vi "RangeFinderCal.vi"() -> ()   [LabVIEW 2014]
uses:
  controls/RangeFind_process.ctl
  controls/ConfigData.ctl
  <vilib>/Instr/_visa.llb/VISA Flush IO Buffer Mask.ctl
  <vilib>/Instr/_visa.llb/VISA Configure Serial Port (Instr).vi
  <vilib>/Utility/file.llb/Write To Spreadsheet File (string).vi
  <vilib>/Analysis/NI_AALBase.lvlib
panel:
  out "Connected":bool
  in  "stop":bool
  in  "Tab Control":T1(tab)
  out "setupEnDisab":bool
  in  "file path (dialog if empty)":path
  in  "Max Range 4":dbl caption="Max Range" format="%.2g"
  in  "Max Range 3":dbl caption="Max Range" format="%.2g"
  in  "Max Range 2":dbl caption="Max Range" format="%.2g"
  in  "Max Range 1":dbl caption="Max Range" format="%.2g"
  in  "Sensor 4 Label":string
  in  "Sensor 3 Label":string
  in  "Sensor 2 Label":string
  in  "Sensor 1 Label":string
  in  "Sample Rate (ms)":dbl=100.0
  in  "Test Name":string
  in  "Connect":bool
  in  "Data System Interface Port":refnum<visa-resource-name>
  out "Range Finder sensor RAW OUTPUT":string
  out "Range Finder sensor parsed output":string[](array[string])
  out "Sensor 4":dbl(slide) caption="Garmin" scale=0.0..200.0
  out "Sensor 3":dbl(slide) caption="HC-SR04" scale=0.0..200.0
  out "Sensor 2":dbl(slide) caption="LidarLite" scale=0.0..200.0
  out "Sensor 1":dbl(slide) caption="SF11-C" scale=0.0..201.0
  in  "Collect":bool
  in  "Comment":string
  out "lblSensor4":string
  out "lblSensor3":string
  out "lblSensor2":string
  out "lblSensor1":string
  in  "Distance":dbl
  out "Mean Sens 4":dbl
  out "S.D. Sensor 4":dbl
  out "Samples":string[][](array[string])
  out "S.D. Sensor 2":dbl
  out "S.D. Sensor 3":dbl
  out "Mean Sens 1":dbl
  out "Mean Sens 2":dbl
  out "Mean Sens 3":dbl
  out "S.D.  Sensor 1":dbl
  in  "writeFile":bool
  out "Activity Log":string
  # ".CSV"
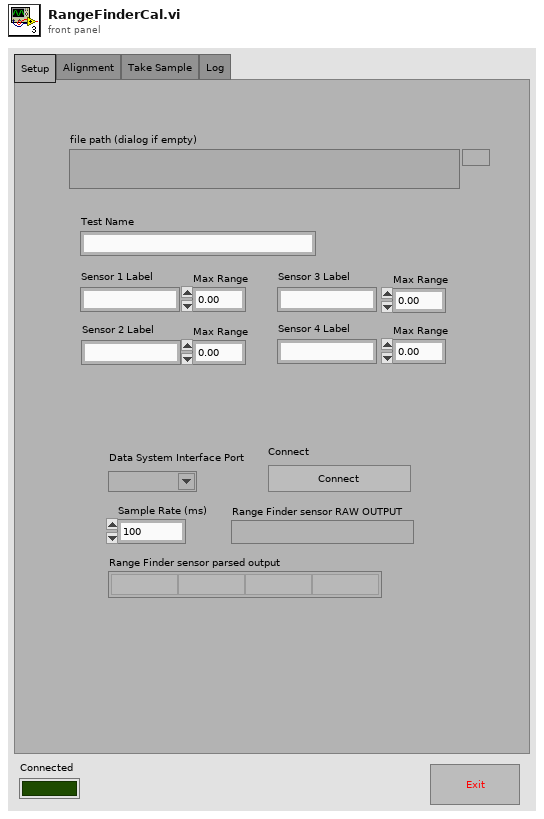
[diagram p1: front panel]
types:
  T1 = enum32{"Setup", "Alignment", "Take Sample", "Log"}
  T2 = typedef "ConfigData.ctl" = cluster{"file path (dialog if empty)":path, "Test Name":string, "Sensor 1 Label":string, "Sensor 2 Label ":string, "Sensor 3 Label":string, "Sensor 4 Label":string, "Max Range":dbl, "Max Range 2":dbl, "Max Range 3":dbl, "Max Range 4":dbl, "Comment":string, "Data System Interface Port":refnum<visa-resource-name>, "Sample Rate":dbl, "error":errorcluster}
  T3 = typedef "RangeFind_process.ctl" = enum16{"Error", "Setup", "Initialize", "Collect", "Store", "Done"}
  T4 = enum8{"Enabled", "Disabled", "Disabled and Grayed Out"}
  T5 = typedef "VISA Flush IO Buffer Mask.ctl" = u16
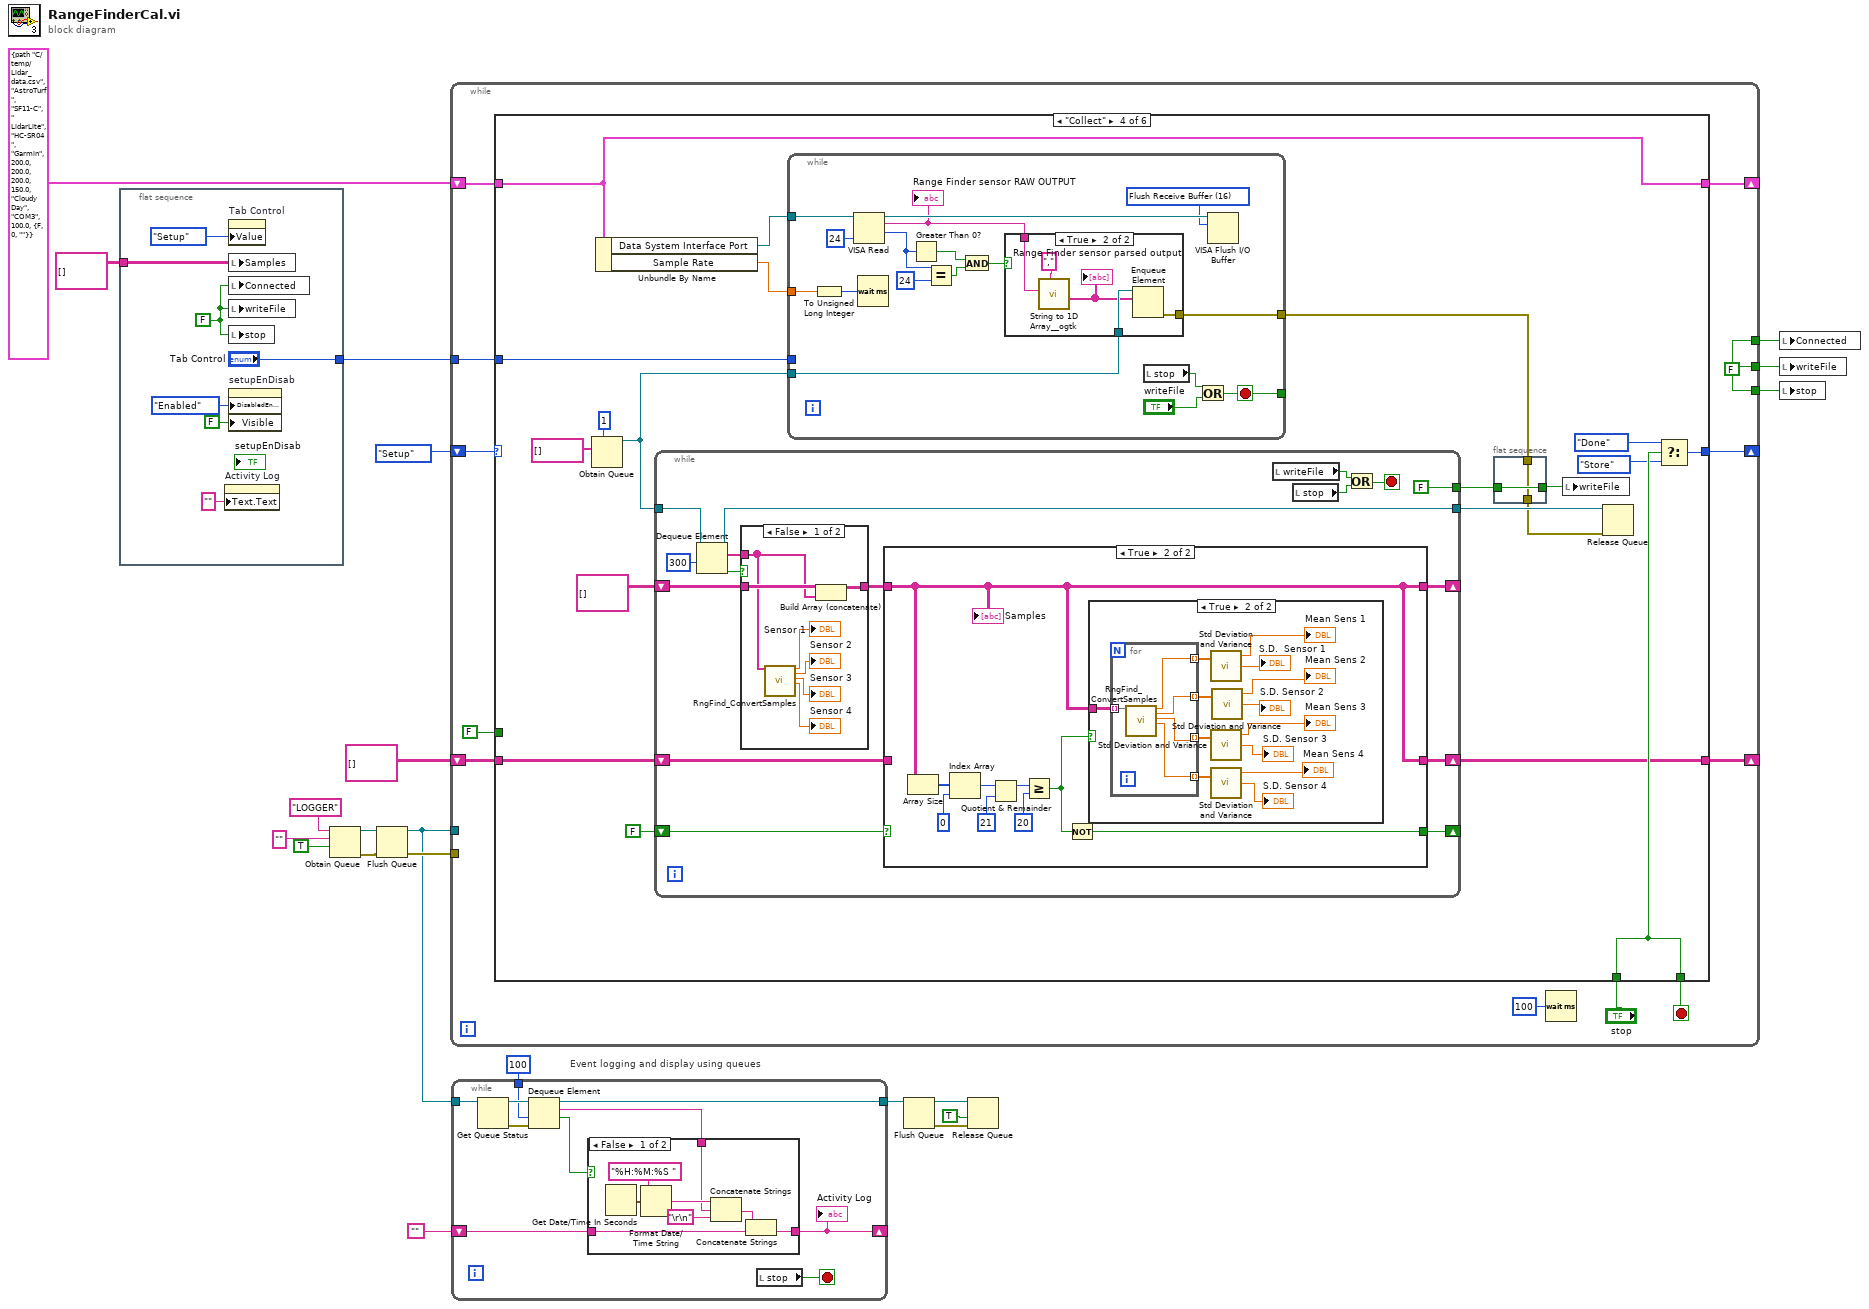
[diagram p0: block diagram]
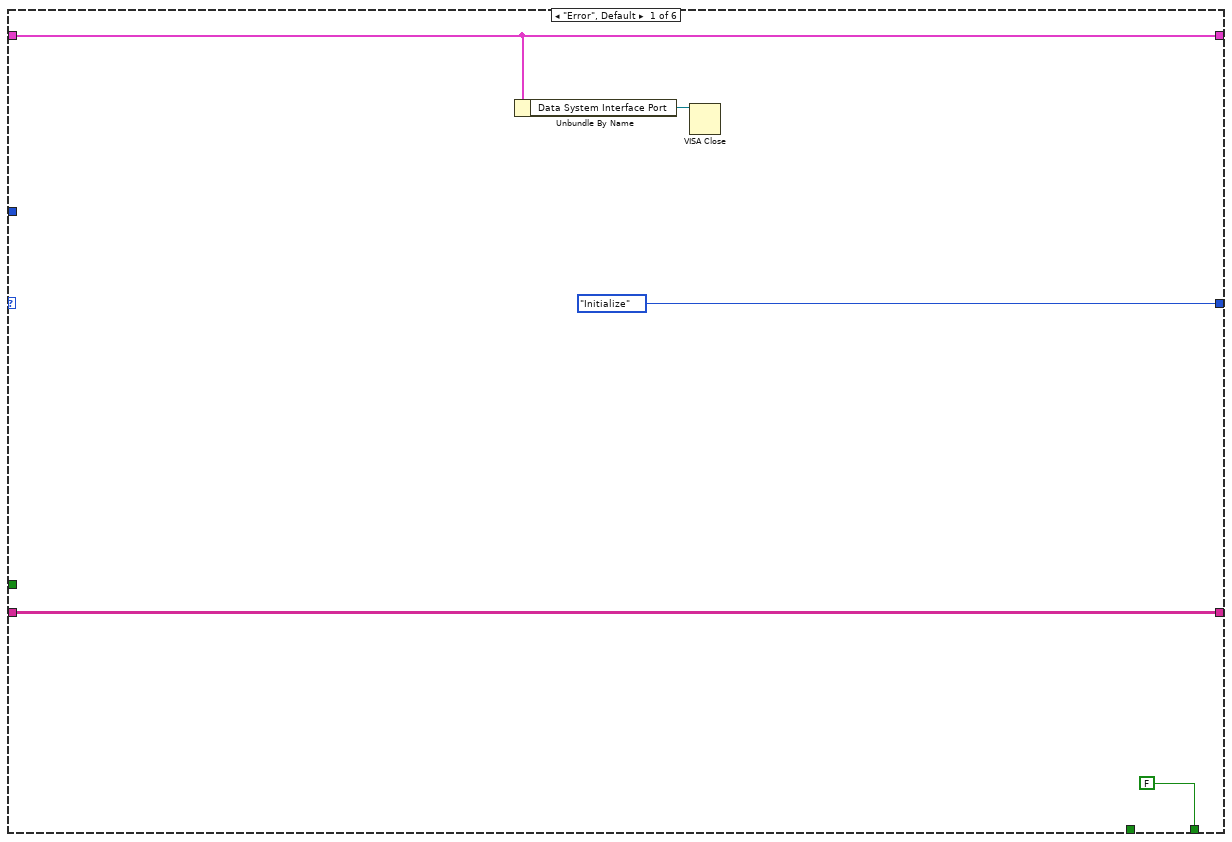
[diagram p3: hidden frame]
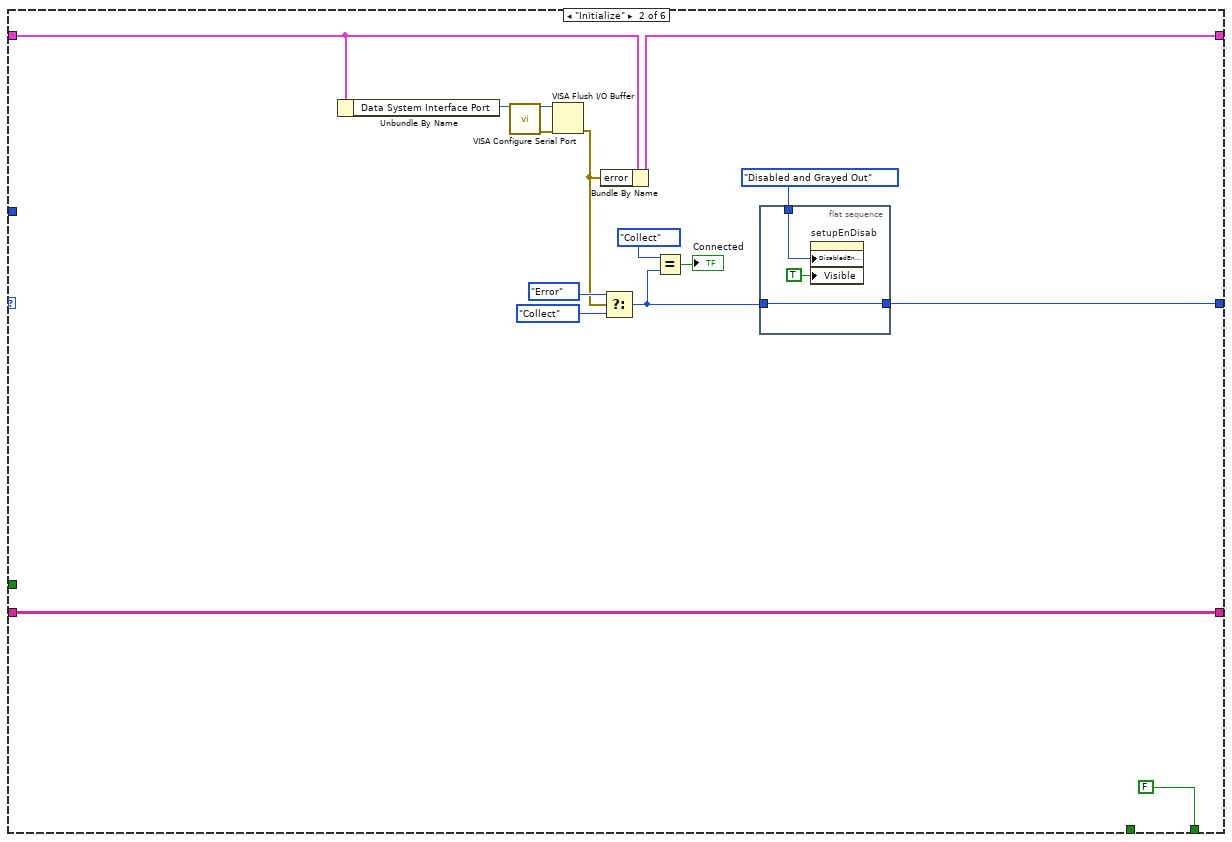
[diagram p4: hidden frame]
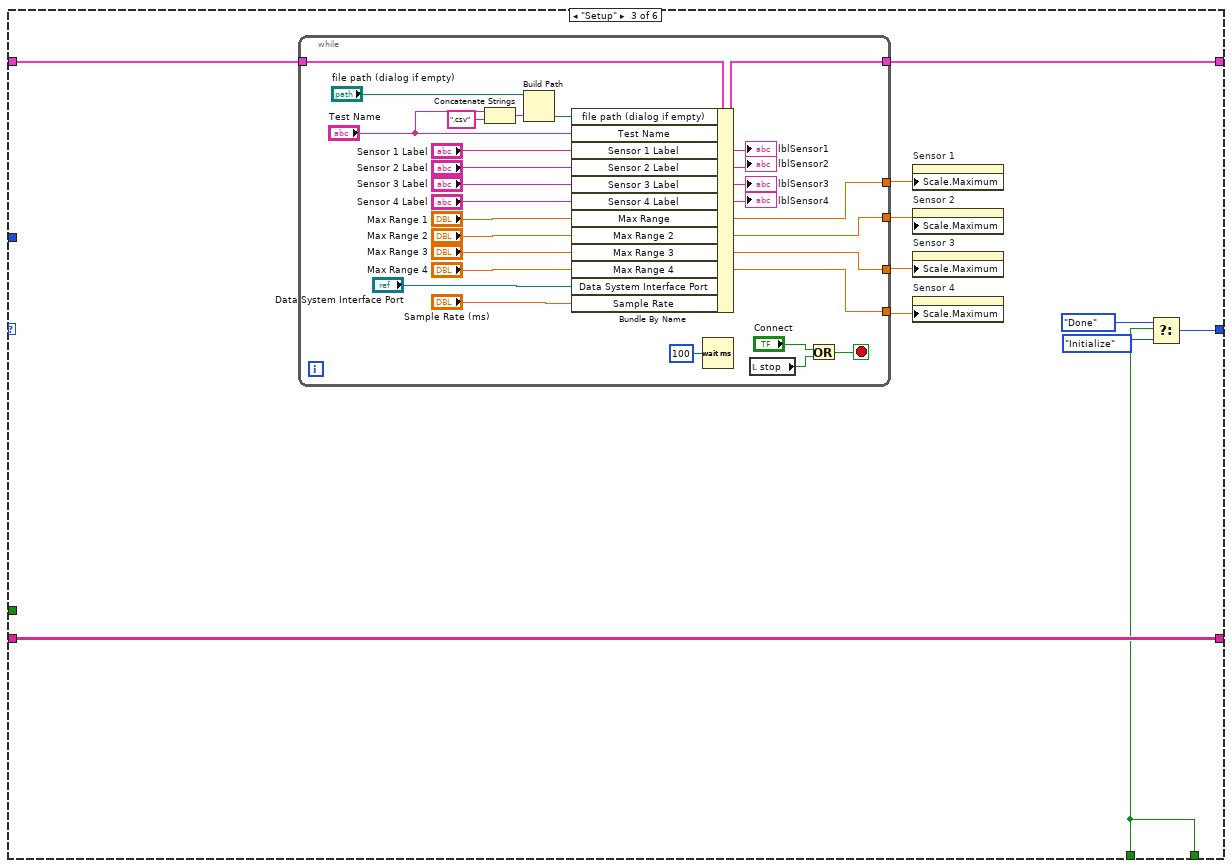
[diagram p5: hidden frame]
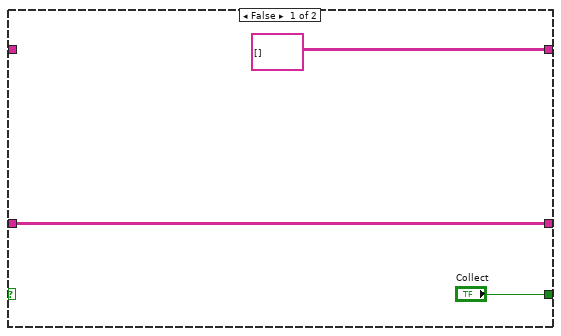
[diagram p6: hidden frame]
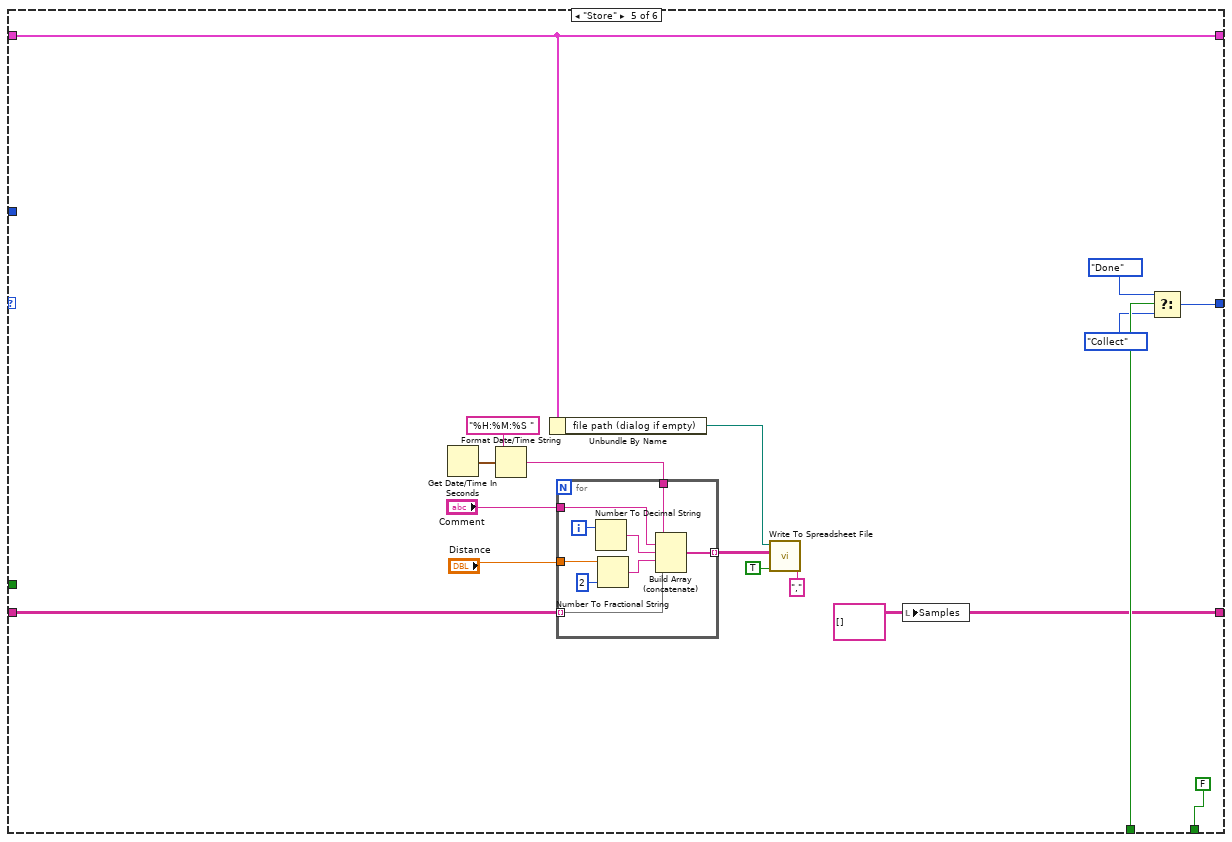
[diagram p10: hidden frame]
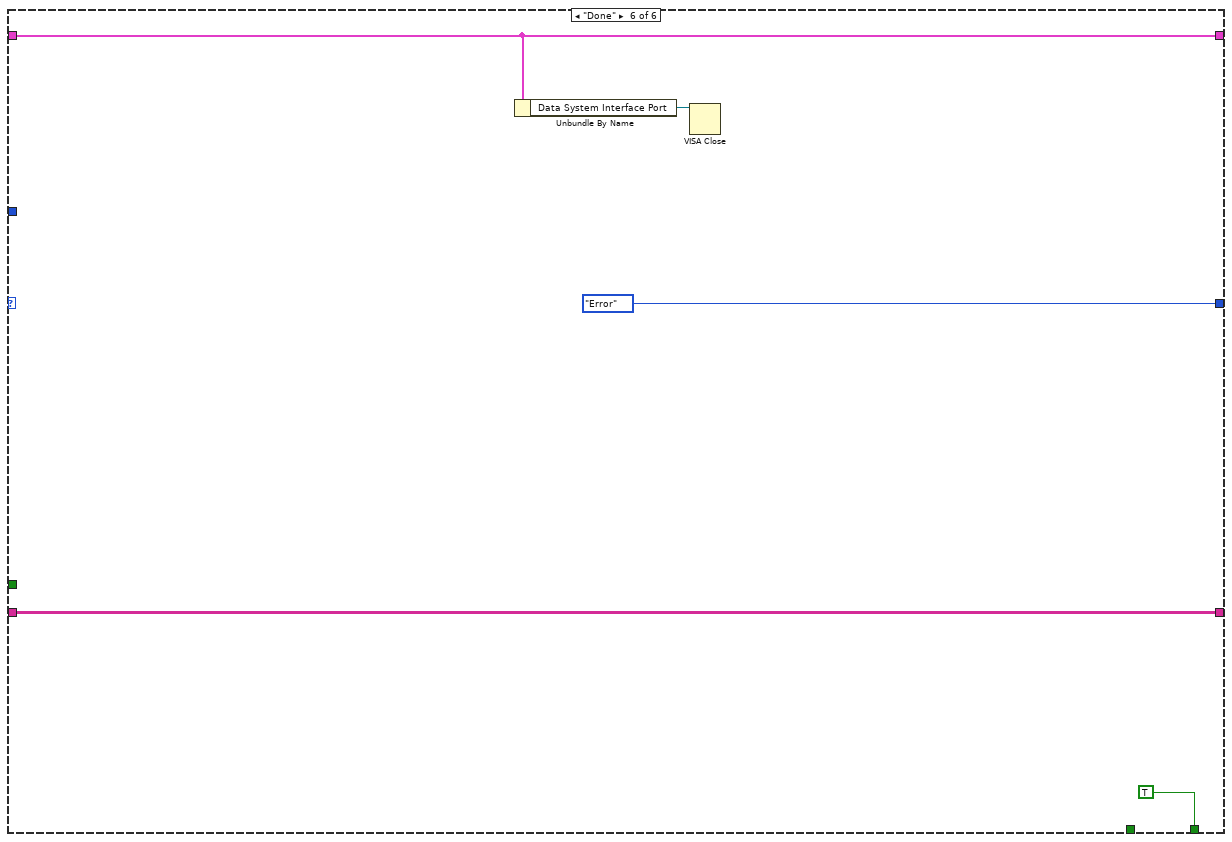
[diagram p11: hidden frame]
diagram:
  # "Event logging and display using queues"
  n1 = flat-sequence {
    tunnel: ["Tab Control"] -> w20
    tunnel: string[][] [] -> [w26]
    frame #0 {
      w25 = FALSE ("stop")
      n2 = property on="Activity Log" class="Str"("Text.Text"="") -> ()  [unwired: 2 in, 2 out]
      n3 = property on="Tab Control" class="TabCtl (strict)"("Value"=T1."Setup" ("Tab Control")) -> ()  [unwired: 2 in, 2 out]
      n4 = local write "Samples"(w26) -> ()
      n5 = local write "Connected"(w25) -> ()
      n6 = local write "writeFile"(w25) -> ()
      n7 = local write "stop"(w25) -> ()
      n8 = property on="setupEnDisab" class="Bool (strict)"("DisabledEnum"=T4."Enabled" ("Disabled"), "Visible"=FALSE) -> ()  [unwired: 2 in, 2 out]
    }
  }
  n9 = Obtain Queue(name (unnamed)="LOGGER", element data type="", create if not found? (T)=TRUE) -> (queue out=w9:refnum<queue>, error out=w13:errorcluster)  [unwired: 2 in, 1 out]
  n10 = Flush Queue(queue=w9) -> (queue out=w3:refnum<queue>)  [unwired: 1 in, 2 out]
  n11 = while {
    tunnel: w20 -> [w39]
    shift-right: [w37] -> _
    shift-left: RangeFind_process."Setup" -> [w38]
    shift-right: [w33] -> _
    shift-left: T2 {"file path (dialog if empty)"=path "C:/temp/Lidar_data.csv", "Test Name"="AstroTurf", "Sensor 1 Label"="SF11-C", "Sensor 2 Label "=" LidarLite", "Sensor 3 Label"="HC-SR04", "Sensor 4 Label"="Garmin", "Max Range"=200.0, "Max Range 2"=200.0, "Max Range 3"=200.0, "Max Range 4"=150.0, "Comment"="Cloudy Day", "Data System Interface Port"="COM3", "Sample Rate"=100.0, "error"={"status"=FALSE, "code"=0, "source"=""}} ("ConfigData") -> [w34]
    shift-right: [w31] -> _
    shift-left: string[][] [] -> [w32]
    tunnel: [w29] -> w16
    tunnel: [w29] -> w15
    tunnel: [w29] -> w14
    tunnel: w13 -> [_]
    tunnel: w3 -> [_]
    stop <- w35 stop-if-true
    w29 = FALSE ("stop")
    n12 = case shown="\"Collect\"" w38 {
      tunnel: w39 -> [_ _ _ w110 _ _]
      tunnel: [RangeFind_process."Initialize" w46 w67 w104 w202 RangeFind_process."Error"] -> w37
      tunnel: [FALSE FALSE w70 w107 FALSE TRUE] -> w35
      tunnel: w34 -> [w40 w52 w73 w108 w207 w219]
      tunnel: [w40 w57 w72 w108 w207 w219] -> w33
      tunnel: w32 -> [w42 w50 w71 w101 w199 w220]
      tunnel: [w42 w50 w71 w103 w200 w220] -> w31
      tunnel: "stop" -> [_ _ w70 w107 w205 _]
      tunnel: FALSE ("stop") -> [_ _ _ _ _ _]
      frame "Error", Default {
        n13 = Unbundle By Name(w40) -> ("Data System Interface Port"=w41:refnum<visa-resource-name>)
        n14 = VISA Close(VISA resource name=w41) -> ()  [unwired: 1 in, 1 out]
      }
      frame "Initialize" {
        n15 = Unbundle By Name(w52) -> ("Data System Interface Port"=w51:refnum<visa-resource-name>)
        n16 = call-poly "VISA Configure Serial Port"("VISA resource name"=w51) -> ("VISA resource name out"=w59:refnum<visa-resource-name>, "error out"=w56:errorcluster)  [unwired: 13 in]
        n17 = VISA Flush I/O Buffer(VISA resource name=w59, error in (no error)=w56) -> (error out=w54:errorcluster)  [unwired: 1 in, 1 out]
        n18 = Bundle By Name(cluster=w52, "error"=w54) -> (w57:T2)
        n19 = Select(t=RangeFind_process."Error", s=w54, f=RangeFind_process."Collect") -> (s? t:f=w47:T3)
        n20 = Equal?(x=RangeFind_process."Collect", y=w47) -> (x = y?=→"Connected":bool)
        n21 = flat-sequence {
          tunnel: w47 -> [w62]
          tunnel: [w62] -> w46
          tunnel: T4."Disabled and Grayed Out" ("Disabled") -> [w60]
          frame #0 {
            n22 = property on="setupEnDisab" class="Bool (strict)"("DisabledEnum"=w60, "Visible"=TRUE) -> ()  [unwired: 2 in, 2 out]
          }
        }
      }
      frame "Setup" {
        n23 = while {
          tunnel: w73 -> [w93]
          tunnel: [w92] -> w72
          tunnel: ["Max Range 1"] -> w66
          tunnel: ["Max Range 2"] -> w65
          tunnel: ["Max Range 3"] -> w64
          tunnel: ["Max Range 4"] -> w63
          stop <- w83 stop-if-true
          n24 = Concatenate Strings("Test Name", ".csv" ("string")) -> (w77:string)
          n25 = Build Path(base path="file path (dialog if empty)", name or relative path=w77) -> (appended path=w76:path)
          n26 = Bundle By Name(cluster=w93, "file path (dialog if empty)"=w76, "Test Name"="Test Name", "Sensor 1 Label"="Sensor 1 Label", "Sensor 2 Label"="Sensor 2 Label", "Sensor 3 Label"="Sensor 3 Label", "Sensor 4 Label"="Sensor 4 Label", "Max Range"="Max Range 1", "Max Range 2"="Max Range 2", "Max Range 3"="Max Range 3", "Max Range 4"="Max Range 4", "Data System Interface Port"="Data System Interface Port", "Sample Rate"="Sample Rate (ms)") -> (w92:T2)
          n27 = Wait (ms)(milliseconds to wait=u32 100) -> ()  [unwired: 1 out]
          n28 = local read "stop"() -> (w84:bool)
          n29 = Or(x="Connect", y=w84) -> (x .or. y?=w83:bool)
          "lblSensor1" <- "Sensor 1 Label"
          "lblSensor2" <- "Sensor 2 Label"
          "lblSensor3" <- "Sensor 3 Label"
          "lblSensor4" <- "Sensor 4 Label"
        }
        n30 = property on="Sensor 1" class="Slide (strict)"("Scale.Maximum"=w66) -> ()  [unwired: 2 in, 2 out]
        n31 = property on="Sensor 2" class="Slide (strict)"("Scale.Maximum"=w65) -> ()  [unwired: 2 in, 2 out]
        n32 = property on="Sensor 3" class="Slide (strict)"("Scale.Maximum"=w64) -> ()  [unwired: 2 in, 2 out]
        n33 = property on="Sensor 4" class="Slide (strict)"("Scale.Maximum"=w63) -> ()  [unwired: 2 in, 2 out]
        n34 = Select(t=RangeFind_process."Done", s=w70, f=RangeFind_process."Initialize") -> (s? t:f=w67:T3)
      }
      frame "Collect" {
        n35 = Obtain Queue(max queue size (-1, unlimited)=1, element data type=string[] []) -> (queue out=w114:refnum<queue>)  [unwired: 3 in, 2 out]
        n36 = Unbundle By Name(w108) -> ("Data System Interface Port"=w109:refnum<visa-resource-name>, "Sample Rate"=w100:dbl)
        n37 = while {
          tunnel: w114 -> [w132]
          tunnel: [w129] -> w112
          shift-right: [w126] -> _
          shift-left: string[][] [] -> [w127]
          tunnel: [FALSE] -> w97
          shift-right: [w119] -> w103
          shift-left: w101 -> [w120]
          shift-right: [w117] -> _
          shift-left: FALSE -> [w118]
          stop <- w121 stop-if-true
          n38 = Dequeue Element(queue=w132, timeout in ms (-1)=300) -> (queue out=w129:refnum<queue>, element=w128:string[], timed out?=w130:bool)  [unwired: 1 in, 1 out]
          n39 = case shown="False" w130 {
            tunnel: w128 -> [w167 _]
            tunnel: w127 -> [w169 w170]
            tunnel: [w168 w170] -> w124
            frame False {
              n40 = call "RngFind_ConvertSamples.vi"("Input Samples"=w167) -> ("sensor 1"=→"Sensor 1":dbl, "sensor 2"=→"Sensor 2":dbl, "sensor 3"=→"Sensor 3":dbl, "sensor 4"=→"Sensor 4":dbl)  [unwired: 15 in]
              n41 = Build Array (concatenate)(w169, w167) -> (w168:string[][])
            }
            frame True {
            }
          }
          n42 = case shown="True" w118 {
            tunnel: [string[][] [] w137] -> w126
            tunnel: w124 -> [_ w137]
            tunnel: w120 -> [w134 _]
            tunnel: [w134 w137] -> w119
            tunnel: ["Collect" w136] -> w117
            frame False {
            }
            frame True {
              n43 = Array Size(array=w137) -> (size(s)=w144:i32[])
              n44 = Index Array(array=w144, index=0) -> (element=w142:i32)
              n45 = Quotient & Remainder(x=w142, y=21) -> (x-y*floor(x/y)=w140:i32)  [unwired: 1 out]
              n46 = Greater Or Equal?(x=w140, y=20) -> (x >= y?=w138:bool)
              n47 = Not(x=w138) -> (.not. x?=w136:bool)
              n48 = case shown="True" w138 {
                tunnel: w137 -> [_ w148]
                frame False {
                }
                frame True {
                  n49 = for {
                    tunnel: w148 -> [w162] mode=indexing
                    tunnel: [w161] -> w157 mode=indexing
                    tunnel: [w158] -> w156 mode=indexing
                    tunnel: [w159] -> w155 mode=indexing
                    tunnel: [w160] -> w147 mode=indexing
                    n50 = call "RngFind_ConvertSamples.vi"("Input Samples"=w162) -> ("sensor 1"=w161:dbl, "sensor 2"=w158:dbl, "sensor 3"=w159:dbl, "sensor 4"=w160:dbl)  [unwired: 15 in]
                  }
                  n51 = call <vilib>:"Std Deviation and Variance.vi"("X"=w157) -> ("mean"=→"Mean Sens 1":dbl, "standard deviation"=→"S.D.  Sensor 1":dbl)  [unwired: 1 in, 1 out]
                  n52 = call <vilib>:"Std Deviation and Variance.vi"("X"=w155) -> ("mean"=→"Mean Sens 3":dbl, "standard deviation"=→"S.D. Sensor 3":dbl)  [unwired: 1 in, 1 out]
                  n53 = call <vilib>:"Std Deviation and Variance.vi"("X"=w147) -> ("mean"=→"Mean Sens 4":dbl, "standard deviation"=→"S.D. Sensor 4":dbl)  [unwired: 1 in, 1 out]
                  n54 = call <vilib>:"Std Deviation and Variance.vi"("X"=w156) -> ("mean"=→"Mean Sens 2":dbl, "standard deviation"=→"S.D. Sensor 2":dbl)  [unwired: 1 in, 1 out]
                }
              }
              "Samples" <- w137
            }
          }
          n55 = local read "writeFile"() -> (w123:bool)
          n56 = local read "stop"() -> (w122:bool)
          n57 = Or(x=w123, y=w122) -> (x .or. y?=w121:bool)
        }
        n58 = while {
          tunnel: w109 -> [w177]
          tunnel: w114 -> [w185]
          tunnel: w110 -> [_]
          tunnel: w100 -> [w182]
          tunnel: [w172] -> _
          tunnel: [w171] -> w98
          stop <- w172 stop-if-true
          w186 = T5 16 items=["Flush Receive Buffer"=16, "Write Transmit Buffer to Device"=32, "Flush Receive Buffer (No I/O)"=64, "Flush Transmit Buffer"=128] ("Mask")
          n59 = To Unsigned Long Integer(number=w182) -> (unsigned 32bit integer=w181:u32)
          n60 = VISA Read(VISA resource name=w177, byte count=u32 24) -> (VISA resource name out=w187:refnum<visa-resource-name>, read buffer=w178:string, return count=w174:u32)  [unwired: 1 in, 1 out]
          "Range Finder sensor RAW OUTPUT" <- w178
          n61 = Wait (ms)(milliseconds to wait=w181) -> ()  [unwired: 1 out]
          n62 = Greater Than 0?(x=w174) -> (x > 0?=w180:bool)
          n63 = Equal?(x=w174, y=u32 24) -> (x = y?=w175:bool)
          n64 = And(x=w180, y=w175) -> (x .and. y?=w179:bool)
          n65 = case shown="True" w179 {
            tunnel: w178 -> [_ w191]
            tunnel: w185 -> [_ w192]
            tunnel: [_ w188] -> w171
            frame False {
            }
            frame True {
              n66 = call <userlib>:"String to 1D Array__ogtk.vi"("delimiter (Tab)"=",", "string"=w191) -> ("Array of Strings"=w189:string[])  [unwired: 9 in]
              "Range Finder sensor parsed output" <- w189
              n67 = Enqueue Element(queue=w192, element=w189) -> (error out=w188:errorcluster)  [unwired: 2 in, 2 out]
            }
          }
          n68 = local read "stop"() -> (w184:bool)
          n69 = Or(x=w184, y="writeFile") -> (x .or. y?=w172:bool)
          n70 = VISA Flush I/O Buffer(VISA resource name=w187, mask (16)=w186) -> ()  [unwired: 1 in, 2 out]
        }
        n71 = flat-sequence {
          tunnel: w98 -> [w115]
          tunnel: w97 -> [w116]
          tunnel: [w116] -> w96
          tunnel: [w115] -> w95
          frame #0 {
          }
        }
        n72 = local write "writeFile"(w96) -> ()
        n73 = Release Queue(queue=w112, error in (no error)=w95) -> ()  [unwired: 1 in, 3 out]
        n74 = Select(t=RangeFind_process."Done", s=w107, f=RangeFind_process."Store") -> (s? t:f=w104:T3)
      }
      frame "Store" {
        w200 = string[][] []
        n75 = Get Date/Time In Seconds() -> (seconds since 1Jan1904=w197:timestamp)
        n76 = Format Date/Time String(time format string (%c)="%H:%M:%S ", seconds (now)=w197) -> (date/time string=w195:string)  [unwired: 1 in]
        n77 = Unbundle By Name(w207) -> ("file path (dialog if empty)"=w206:path)
        n78 = for {
          tunnel: w199 -> [w215] mode=indexing
          tunnel: "Distance" -> [w218]
          tunnel: [w217] -> w193 mode=indexing
          tunnel: w195 -> [w211]
          tunnel: "Comment" -> [w210]
          i -> [w213]
          n79 = Number To Decimal String(number=w213) -> (decimal integer string=w212:string)  [unwired: 1 in]
          n80 = Number To Fractional String(number=w218, precision (6)=i16 2) -> (F-format string=w214:string)  [unwired: 2 in]
          n81 = Build Array (concatenate)(w211, w210, w212, w214, w215) -> (w217:string[])
        }
        n82 = call-poly <vilib>:"Write To Spreadsheet File.vi"("delimiter (\\t)"="," ("delimiter (\\t)"), "append to file? (new file:F)"=TRUE, "2D data"=w193, "file path (dialog if empty)"=w206) -> ()  [unwired: 4 in, 1 out]
        n83 = local write "Samples"(w200) -> ()
        n84 = Select(t=RangeFind_process."Done", s=w205, f=RangeFind_process."Collect") -> (s? t:f=w202:T3)
      }
      frame "Done" {
        n85 = Unbundle By Name(w219) -> ("Data System Interface Port"=w221:refnum<visa-resource-name>)
        n86 = VISA Close(VISA resource name=w221) -> ()  [unwired: 1 in, 1 out]
      }
    }
    n87 = Wait (ms)(milliseconds to wait=u32 100) -> ()  [unwired: 1 out]
  }
  n88 = while {
    tunnel: w3 -> [w233]
    shift-right: [w224] -> _
    shift-left: "" -> [w226]
    tunnel: [w232] -> w8
    tunnel: 100 ("timeout in ms (-1)") -> [w225]
    stop <- w229 stop-if-true
    n89 = Get Queue Status(queue=w233) -> (queue out=w231:refnum<queue>, error out=w230:errorcluster)  [unwired: 2 in, 6 out]
    n90 = Dequeue Element(queue=w231, timeout in ms (-1)=w225, error in (no error)=w230) -> (queue out=w232:refnum<queue>, element=w227:string, timed out?=w228:bool)  [unwired: 1 out]
    n91 = case shown="False" w228 {
      tunnel: w227 -> [w234 _]
      tunnel: w226 -> [w236 w242]
      tunnel: [w235 w242] -> w224
      frame False {
        n92 = Get Date/Time In Seconds() -> (seconds since 1Jan1904=w239:timestamp)
        n93 = Format Date/Time String(time format string (%c)="%H:%M:%S ", seconds (now)=w239) -> (date/time string=w238:string)  [unwired: 1 in]
        n94 = Concatenate Strings(w238, w234, "\r\n") -> (w241:string)
        n95 = Concatenate Strings(w241, w236) -> (w235:string)
      }
      frame True {
      }
    }
    "Activity Log" <- w224
    n96 = local read "stop"() -> (w229:bool)
  }
  n97 = Flush Queue(queue=w8) -> (queue out=w6:refnum<queue>, error out=w5:errorcluster)  [unwired: 1 in, 1 out]
  n98 = Release Queue(queue=w6, force destroy? (F)=TRUE, error in (no error)=w5) -> ()  [unwired: 3 out]
  n99 = local write "Connected"(w14) -> ()
  n100 = local write "writeFile"(w16) -> ()
  n101 = local write "stop"(w15) -> ()
